vi "finishSimplePassPlay.vi"(8 "error in (no error)":errorcluster, 10 "Game in":refnum<class "Game.lvclass">, 11 "SimplePass in":refnum<class "SimplePass.lvclass">) -> (0 "error out":errorcluster, 2 "finishSimplePass?":bool, 3 "SimplePass out":refnum<class "SimplePass.lvclass">)   [LabVIEW 2023, in "SimplePass.lvclass"]
uses:
  SimplePass.lvclass
  Game_class/Game.lvclass
  Referee_class/command_interpreted.ctl
  Game_class/Game.lvclass/Game.ctl
  Referee_class/Referee.lvclass/Referee.ctl
  Events_class/Events.lvclass/Events.ctl
  Team_class/Team.lvclass/Team.ctl
  Game_class/Read Referee.vi
  Game_class/Read EventsRef.vi
  Game_class/Read OffensiveTeam.vi
  Team_class/Read OffensivePlay Finished.vi
  Events_class/Read ball_out.vi
  Referee_class/Read command_interpreted.vi
  Ally_class/Ally.lvclass
  Referee_class/Referee.lvclass
  Events_class/Events.lvclass
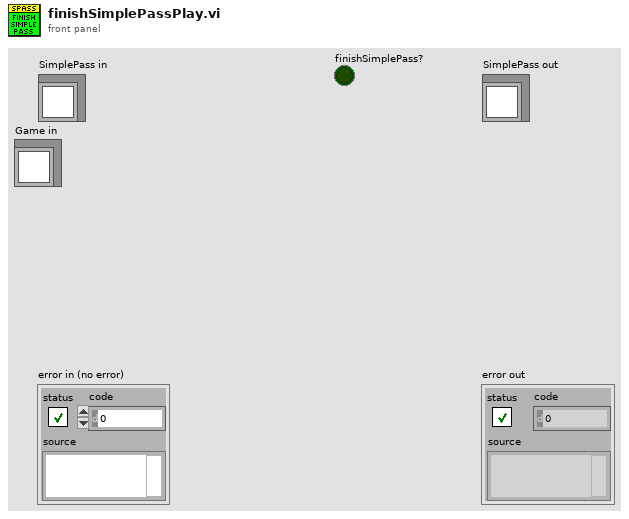
[diagram p1: front panel]
types:
  T1 = typedef "command_interpreted.ctl" = enum16{"Goal Ally", "Goal Enemy", "Ball Placement Enemy", "Ball Placement Ally", "Normal Half Time", "Extra Time  Break", "Extra Half Time", "None", "Post Game", "PKA Normal Start", "Prepare Kickoff Ally", "PKE Normal Start", "Prepare Kickoff Enemy", "Force Start", "Halt", "Timeout", "Prepare Penalty Ally", "Prepare Penalty Enemy", "PPA NormalStart", "PPE Normal Start", "Indirect Free Ally", "Direct Free Enemy", "Direct Free Ally", "Indirect Free Enemy", "Stop"}
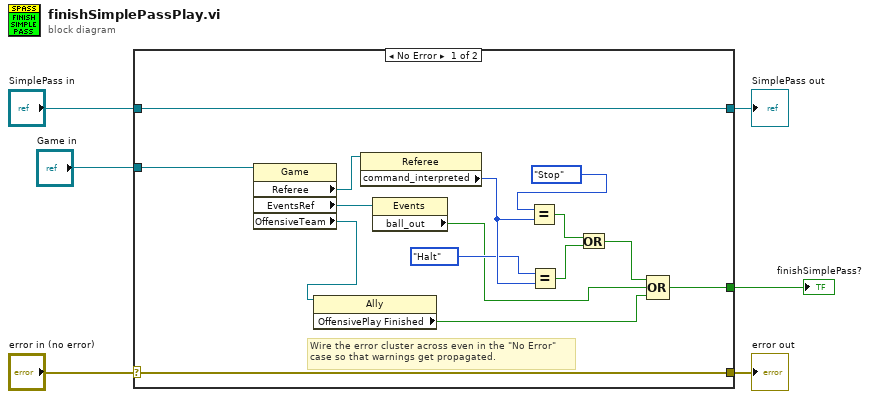
[diagram p0: block diagram]
diagram:
  n1 = case shown="No Error" "error in (no error)" {
    selector: "error in (no error)" -> [w20 w23]
    tunnel: [w20 w23] -> w5
    tunnel: [w21 w22] -> w3
    tunnel: "SimplePass in" -> [w21 w22]
    tunnel: "Game in" -> [w8 _]
    tunnel: [w7 _] -> w1
    frame No Error {
      # "Wire the error cluster across even in the \"No Error\"\ncase so that warnings get propagated."
      n2 = property class="Game"(reference=w8) -> ("Referee"=w19:refnum<class "Referee.lvclass">, "EventsRef"=w18:refnum<class "Events.lvclass">, "OffensiveTeam"=w17:refnum<class "Ally.lvclass">)  [unwired: 1 in, 2 out]
      n3 = property class="Ally"(reference=w17) -> ("OffensivePlay Finished"=w9:bool)  [unwired: 1 in, 2 out]
      n4 = property class="Referee"(reference=w19) -> ("command_interpreted"=w15:T1)  [unwired: 1 in, 2 out]
      n5 = property class="Events"(reference=w18) -> ("ball_out"=w10:bool)  [unwired: 1 in, 2 out]
      n6 = Equal?(x=command_interpreted."Stop" ("command_interpreted"), y=w15) -> (x = y?=w13:bool)
      n7 = Equal?(x=command_interpreted."Halt" ("command_interpreted"), y=w15) -> (x = y?=w12:bool)
      n8 = Or(x=w13, y=w12) -> (x .or. y?=w11:bool)
      n9 = Compound Arithmetic op=OR(w11, w10, w9) -> (w7:bool)
    }
    frame Error {
    }
  }
  "error out" <- w5
  "SimplePass out" <- w3
  "finishSimplePass?" <- w1
